vi "State1-Drive.vi"(9 "Boolean":bool) -> (1 "Left/Right":enum16{"Left", "Right", "Stop"}(ring), 2 "Front/Back 2":enum16{"Forward", "Backward", "Stop"}(ring), 3 "Front/Back Speed":u32, 4 "Left/Right Speed":u32, 5 "Enum":T1, 6 "Cluster":T2)   [LabVIEW 2014]
uses:
  FPGA Bitfiles/Parking States Indicators.ctl
  FPGA Bitfiles/Parking States.ctl
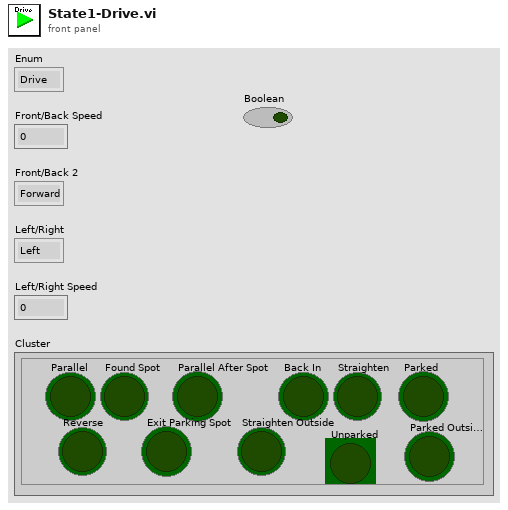
[diagram p1: front panel]
types:
  T1 = typedef "Parking States.ctl" = enum16{"Drive", "Parallel", "Found Spot", "Parallel After Spot", "Back In", "Straighten", "Parked", "Reverse", "Exit Parking Spot", "Straighten Outside", "Unparked", "Parked Outside"}
  T2 = typedef "Parking States Indicators.ctl" = cluster{"Parallel":bool, "Found Spot":bool, "Parallel After Spot":bool, "Back In":bool, "Straighten":bool, "Parked":bool, "Reverse":bool, "Exit Parking Spot":bool, "Straighten Outside":bool, "Unparked":bool, "Parked Outside":bool}
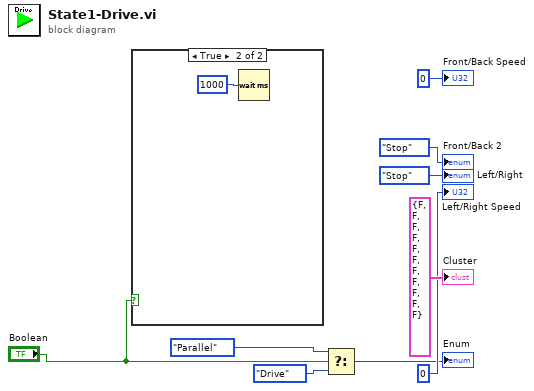
[diagram p0: block diagram]
diagram:
  n1 = case shown="True" "Boolean" {
    frame False {
    }
    frame True {
      n2 = Wait (ms)(milliseconds to wait=u32 1000) -> ()  [unwired: 1 out]
    }
  }
  n3 = Select(t=Parking_States."Parallel", s="Boolean", f=Parking_States."Drive") -> (s? t:f=→"Enum":T1)
  "Cluster" <- T2 {"Parallel"=FALSE, "Found Spot"=FALSE, "Parallel After Spot"=FALSE, "Back In"=FALSE, "Straighten"=FALSE, "Parked"=FALSE, "Reverse"=FALSE, "Exit Parking Spot"=FALSE, "Straighten Outside"=FALSE, "Unparked"=FALSE, "Parked Outside"=FALSE} ("Cluster")
  "Front/Back Speed" <- u32 0 ("Front/Back Speed")
  "Front/Back 2" <- enum16{"Forward", "Backward", "Stop"}."Stop" ("Front/Back 2")
  "Left/Right" <- enum16{"Left", "Right", "Stop"}."Stop" ("Left/Right")
  "Left/Right Speed" <- u32 0 ("Left/Right Speed")
